vi "Get Sensor Values.vi"(11 "Motors":T2) -> (0 "Steer Angles (ticks)":T1, 1 "Drive Velocities (ticks/ds)":T1, 2 "Steer Angles (degrees)":T1, 3 "Drive Velocities (ft/s)":T1)   [LabVIEW 2020]
doc: "Gets sensor velocities and positions from the pods"
uses:
  ctl/Swerve Motors.ctl
  ctl/4 Motor Set.ctl
  <vilib>/Rock Robotics/WPI/MotorControl/WPI_MotorControlDeviceRef.ctl
  <vilib>/Rock Robotics/WPI/MotorControl/WPI_MotorControlType.ctl
  <vilib>/Rock Robotics/SystemInterfaces/DIO/FPGA_DIOPWMChannel.ctl
  <vilib>/Rock Robotics/WPI/PWM/WPI_PWMDeadband.ctl
  <vilib>/Rock Robotics/SystemInterfaces/DIO/FPGA_DIOChannel.ctl
  <vilib>/Rock Robotics/WPI/ThirdParty/Phoenix-LabVIEW/Motor Controller/Get/CTRE_Phoenix_MotorController_GetSelectedSensorData.vi
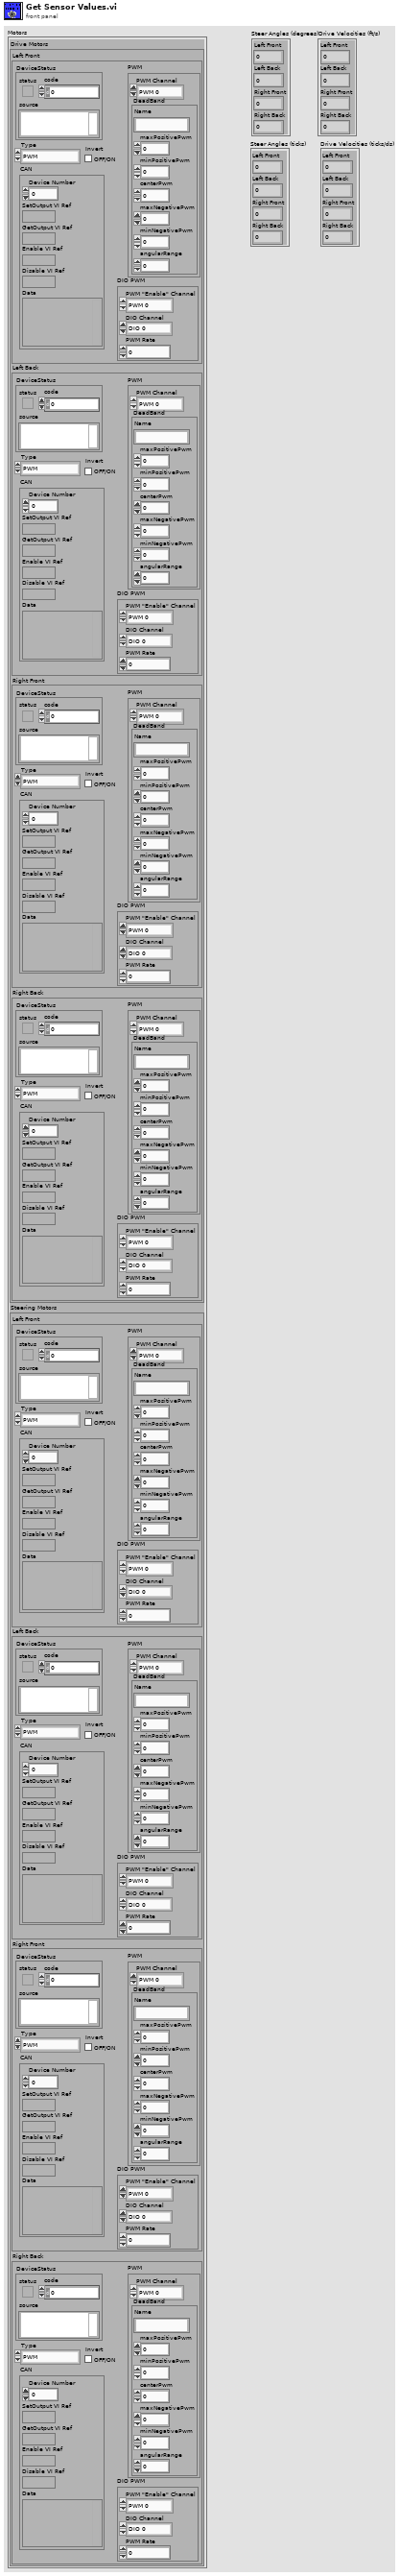
[diagram p1: front panel]
types:
  T1 = cluster{"Left Front":i32, "Left Back":i32, "Right Front":i32, "Right Back":i32}
  T2 = typedef "Swerve Motors.ctl" = cluster{"Drive Motors":T3, "Steering Motors":T3}
  T3 = typedef "4 Motor Set.ctl" = cluster{"Left Front":T4, "Left Back":T4, "Right Front":T4, "Right Back":T4}
  T4 = typedef "WPI_MotorControlDeviceRef.ctl" = cluster{"DeviceStatus":errorcluster, "Type":T5, "PWM":cluster{"PWM Channel":T6, "DeadBand":T7}, "CAN":cluster{"Device Number":u8, "SetOutput VI Ref":variant, "GetOutput VI Ref":variant, "Enable VI Ref":variant, "Disable VI Ref":variant, "Data":variant}, "Invert":bool, "DIO PWM":cluster{"PWM \"Enable\" Channel":T6, "DIOChannel":T8, "PWM Rate":dbl}}
  T5 = typedef "WPI_MotorControlType.ctl" = enum16{"PWM", "CAN", "DIO PWM"}
  T6 = typedef "FPGA_DIOPWMChannel.ctl" = enum8{"PWM 0", "PWM 1", "PWM 2", "PWM 3", "PWM 4", "PWM 5", "PWM 6", "PWM 7", "PWM 8", "PWM 9", "PWM MXP 0", "PWM MXP 1", "PWM MXP 2", "PWM MXP 3", "PWM MXP 4", "PWM MXP 5", "PWM MXP 6", "PWM MXP 7", "PWM MXP 8", "PWM MXP 9", "Invalid"}
  T7 = typedef "WPI_PWMDeadband.ctl" = cluster{"Name":string, "maxPositivePwm":i32, "minPositivePwm":i32, "centerPwm":i32, "maxNegativePwm":i32, "minNegativePwm":i32, "angularRange":u16}
  T8 = typedef "FPGA_DIOChannel.ctl" = enum8{"DIO 0", "DIO 1", "DIO 2", "DIO 3", "DIO 4", "DIO 5", "DIO 6", "DIO 7", "DIO 8", "DIO 9", "DIO MXP 0", "DIO MXP 1", "DIO MXP 2", "DIO MXP 3", "DIO MXP 4", "DIO MXP 5", "DIO MXP 6", "DIO MXP 7", "DIO MXP 8", "DIO MXP 9", "DIO MXP 10", "DIO MXP 11", "DIO MXP 12", "DIO MXP 13", "DIO MXP 14", "DIO MXP 15", "SPI Port CS1", "SPI Port CS2", "SPI Port CS3", "SPI Port MISO", "SPI Port MOSI", "Invalid"}
  T9 = cluster{"[0]":i32, "[1]":i32, "[2]":i32, "[3]":i32}
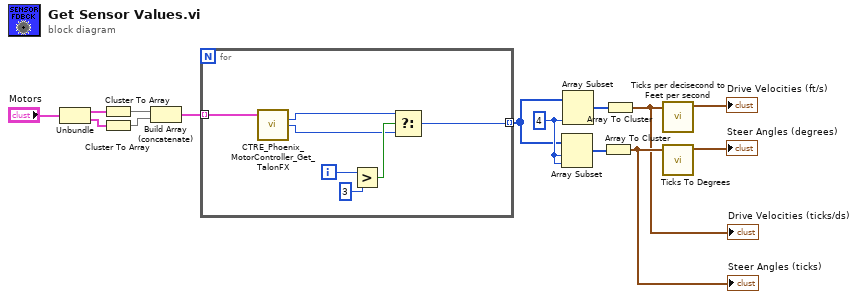
[diagram p0: block diagram]
diagram:
  w8 = 4 ("length")
  n1 = Unbundle("Motors") -> ("Drive Motors"=w13:T3, "Steering Motors"=w12:T3)
  n2 = Cluster To Array(cluster=w13) -> (array=w11:T4[])
  n3 = Cluster To Array(cluster=w12) -> (array=w10:T4[])
  n4 = Build Array (concatenate)(w11, w10) -> (w9:T4[])
  n5 = for {
    tunnel: w9 -> [w19] mode=indexing
    tunnel: [w15] -> w7 mode=indexing
    i -> [w21]
    n6 = call-poly <vilib>:"CTRE_Phoenix_MotorController_Get_TalonFX.vi"("PhoenixMotorControlDevRef"=w19) -> ("Position (Raw Sensor Units)"=w17:i32, "Velocity (Raw Sensor Units per 100 ms)"=w16:i32)  [unwired: 11 in, 2 out]
    n7 = Greater?(x=w21, y=3) -> (0:w18:bool)
    n8 = Select(t=w17, s=w18, f=w16) -> (s? t:f=w15:i32)
  }
  n9 = Array Subset(array=w7, index=w8, length=w8) -> (w5:i32[])
  n10 = Array Subset(array=w7, length=w8) -> (w6:i32[])  [unwired: 1 in]
  n11 = Array To Cluster(array=w5) -> (cluster=w4:T9)
  "Steer Angles (ticks)" <- w4
  n12 = Array To Cluster(array=w6) -> (cluster=w3:T9)
  "Drive Velocities (ticks/ds)" <- w3
  n13 = call "Ticks per decisecond to Feet per second.vi"("Drive Velocities (ticks/ds)"=w3) -> ("Drive Velocities (ft/s)"=→"Drive Velocities (ft/s)":T1)  [unwired: 10 in]
  n14 = call "Ticks To Degrees.vi"("Steer Angles (ticks)"=w4) -> ("Steer Angles (degrees)"=→"Steer Angles (degrees)":T1)  [unwired: 10 in]
